vi "Configure OSC Limit Open query.vi"(7 "Mode":T1 items=["OSC"], 8 "error in (no error)":errorcluster, 10 "Step":T2=1 min=1 max=99 step=1, 11 "VISA resource name":refnum<visa-resource-name>) -> (0 "error out":errorcluster, 2 "Limit open":string, 3 "VISA resource name out":refnum<visa-resource-name>)   [LabVIEW 2025]
uses:
  <instrlib>/Chroma 19052/Public/Utility/Type Def/steps--numeric.ctl
  <instrlib>/Chroma 19052/Public/Utility/Type Def/OSC mode--ring.ctl
  <instrlib>/Chroma 19052/Chroma 19052.lvlib
panel:
  # "OSC Limit Open query"
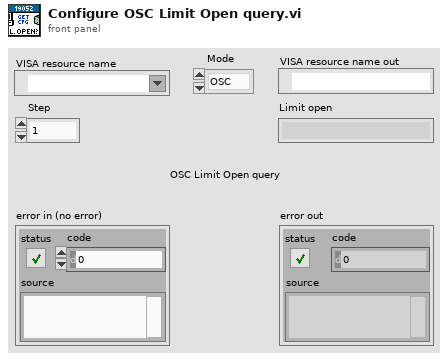
[diagram p1: front panel]
types:
  T1 = typedef "Chroma 19052.lvlib/OSC mode--ring.ctl" = i32
  T2 = typedef "Chroma 19052.lvlib/steps--numeric.ctl" = u8
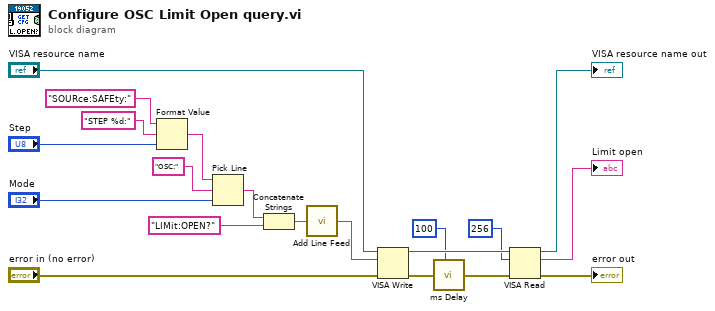
[diagram p0: block diagram]
diagram:
  n1 = Format Value(string ("")="SOURce:SAFEty:", format string="STEP %d:", value (0)="Step") -> (output string=w16:string)
  n2 = Pick Line(string ("")=w16, multi-line string="OSC:", line index="Mode") -> (output string=w12:string)
  n3 = Concatenate Strings(w12, "LIMit:OPEN?" ("format string")) -> (w10:string)
  n4 = call <instrlib>:"Add Line Feed.vi"("Command string"=w10) -> ("Concatenated string"=w8:string)  [unwired: 4 in]
  n5 = VISA Write(VISA resource name="VISA resource name", write buffer=w8, error in (no error)="error in (no error)") -> (VISA resource name out=w20:refnum<visa-resource-name>, error out=w5:errorcluster)  [unwired: 1 out]
  n6 = call <instrlib>:"ms Delay.vi"("miliseconds to wait"=u32 100 ("Time Delay ms"), "error in (no error)"=w5) -> ("error out"=w4:errorcluster)  [unwired: 6 in, 1 out]
  n7 = VISA Read(VISA resource name=w20, byte count=u32 256, error in (no error)=w4) -> (VISA resource name out=→"VISA resource name out":refnum<visa-resource-name>, read buffer=→"Limit open":string, error out=→"error out":errorcluster)  [unwired: 1 out]
